vi "Merge Two Images.vi"(2 "Set Background Color (T)":bool=TRUE, 4 "Image 2 Bounds":T1={"Left"=0, "Top"=0, "Right"=64, "Bottom"=64}, 5 "Image 2 Data":T2, 6 "Image 1 Bounds":T1={"Left"=0, "Top"=0, "Right"=64, "Bottom"=64}, 7 "Image 1 Data":T2, 8 "error in (no error)":errorcluster, 9 "Background Color":u32(colorbox)=16777215, 10 "Image 2 Path":path, 11 "Image 1 Path":path) -> (0 "error out":errorcluster, 3 "Merged Image Data":T2)   [LabVIEW 2015]
doc: "This VI will merge two images into one. This merge supports PNGs and GIFs with alpha layers. Provide the path to <B>Image 1 Path</B> and <B>Image 2 Path</B> or provide the <B>Image 1 Data</B> and <B>Image 2 Data</B> or a combination of the two. Then provide the scaled <B>Image Bounds</B> and <B>Image 2 Bounds</B>. The output image will be large enough to contain both images. If both images have an alpha layer, then the <B>Background Color</B> should be provided.\n\n-------------\nDeveloped by Brian Hoover (hooovahh)"
uses:
  <vilib>/picture/picture.llb/imagedata.ctl
  <vilib>/Utility/miscctls.llb/LVRectTypeDef.ctl
  System.Drawing
  <vilib>/wsapi/NI_WebServices.lvlib
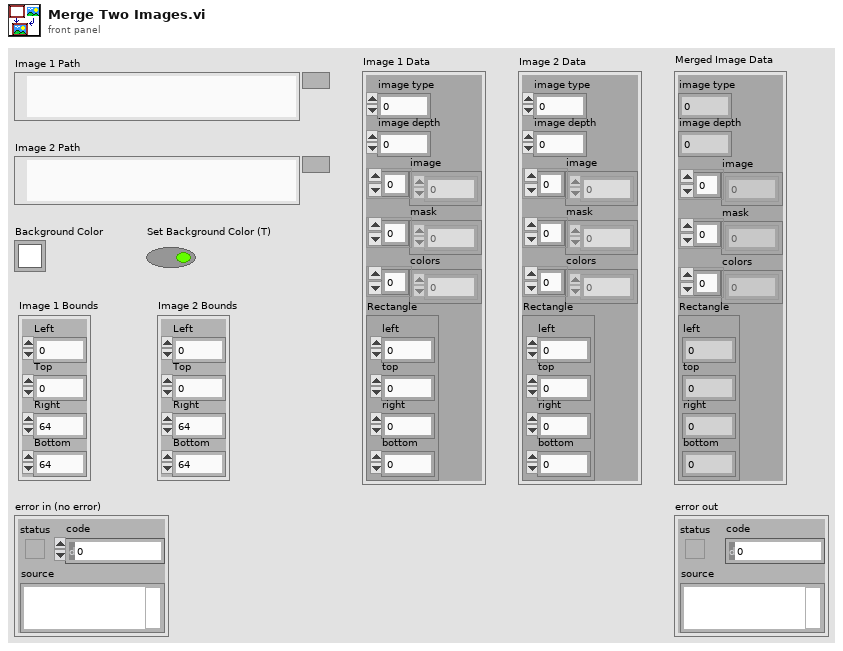
[diagram p1: front panel]
types:
  T1 = typedef "LVRectTypeDef.ctl" = cluster{"Left":i16, "Top":i16, "Right":i16, "Bottom":i16}
  T2 = typedef "imagedata.ctl" = cluster{"image type":i32, "image depth":i32, "image":u8[], "mask":u8[], "colors":u32[], "Rectangle":cluster{"left":i16, "top":i16, "right":i16, "bottom":i16}}
  T3 = typedef "LVBoundsTypeDef.ctl" = cluster{"Width":u32, "Height":u32}
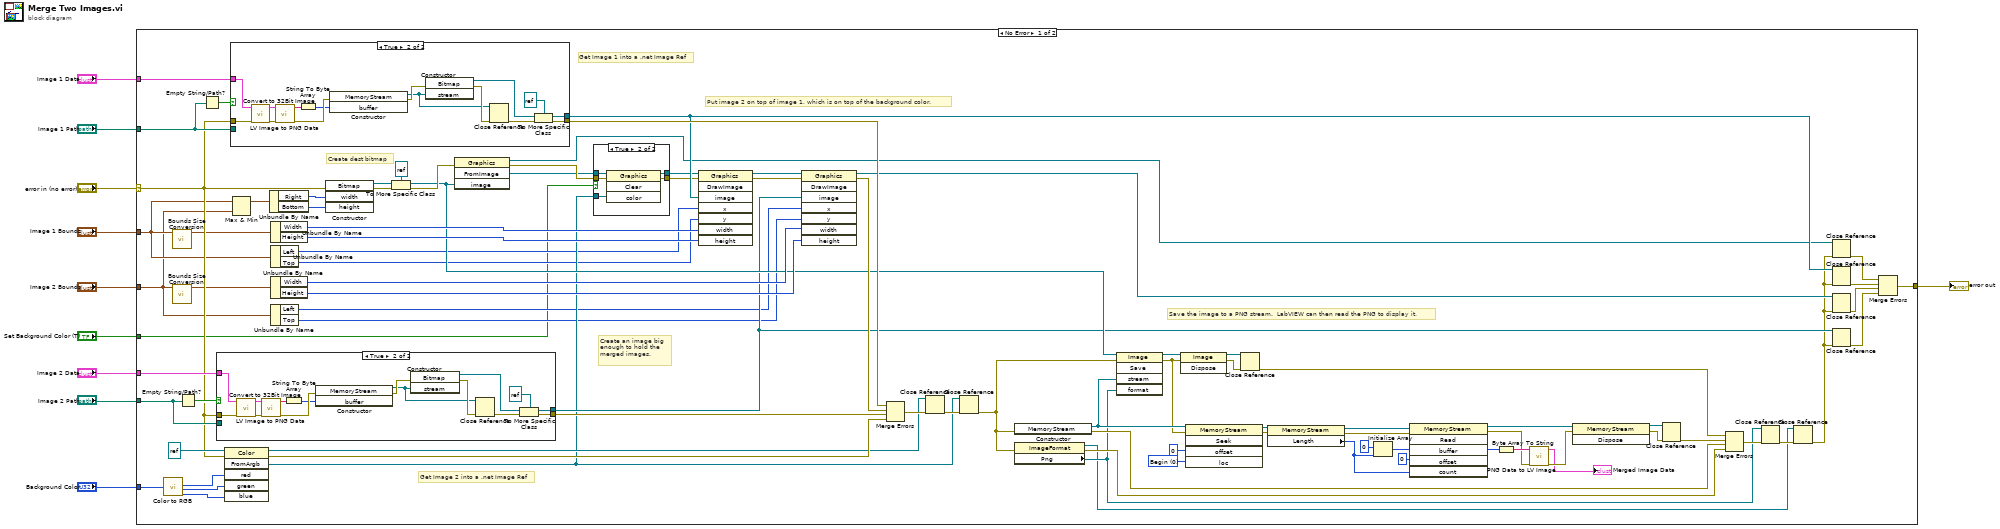
[diagram p0: block diagram]
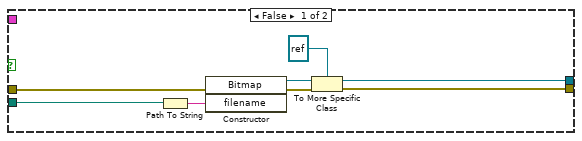
[diagram p3: hidden frame]
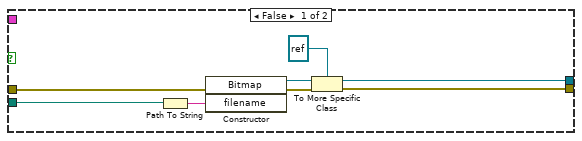
[diagram p4: hidden frame]
diagram:
  n1 = case shown="No Error" "error in (no error)" {
    selector: "error in (no error)" -> [w21 w153]
    tunnel: [w77 w153] -> w10
    tunnel: "Background Color" -> [w46 _]
    tunnel: "Image 1 Path" -> [w42 _]
    tunnel: "Image 1 Data" -> [w40 _]
    tunnel: "Image 2 Path" -> [w37 _]
    tunnel: "Image 2 Data" -> [w36 _]
    tunnel: "Image 1 Bounds" -> [w14 _]
    tunnel: "Image 2 Bounds" -> [w13 _]
    tunnel: "Set Background Color (T)" -> [w11 _]
    frame No Error {
      w69 = 0 items=["Begin", "Current", "End"] ("loc")
      # "Save the image to a PNG stream.  LabVIEW can then read the PNG to display it."
      # "Put image 2 on top of image 1, which is on top of the background color."
      # "Create an image big enough to hold the merged images."
      # "Get Image 1 into a .net Image Ref"
      # "Get Image 2 into a .net Image Ref"
      # "Create dest bitmap"
      n2 = call <vilib>:"Color to RGB.vi"("Color"=w46) -> ("R"=w45:u8, "G"=w44:u8, "B"=w43:u8)  [unwired: 1 out]
      n3 = call "Bounds Size Conversion.vi"("Bounds"=w14) -> ("Size Out"=w19:T3)  [unwired: 9 in, 1 out]
      n4 = call "Bounds Size Conversion.vi"("Bounds"=w13) -> ("Size Out"=w20:T3)  [unwired: 9 in, 1 out]
      n5 = Empty String/Path?(string/path=w37) -> (empty?=w38:bool)
      n6 = Empty String/Path?(string/path=w42) -> (empty?=w41:bool)
      n7 = case shown="True" w38 {
        tunnel: w21 -> [w110 w124]
        tunnel: w37 -> [w109 _]
        tunnel: [w108 w118] -> w35
        tunnel: [w107 w116] -> w39
        tunnel: w36 -> [_ w123]
        frame False {
          n8 = Path To String(path=w109) -> (string=w114:string)
          n9 = constructor class="Bitmap"(error in=w110, "filename"=w114) -> (reference out=w112:refnum<k24>, error out=w111:errorcluster)  [unwired: 2 in, 2 out]
          n10 = To More Specific Class(target class=refnum<k24> refnum, reference=w112, error in=w111) -> (specific class reference=w107:refnum<k24>, error out=w108:errorcluster)
        }
        frame True {
          n11 = call "Convert to 32Bit Image.vi"("error in (no error)"=w124, "Image Data"=w123) -> ("error out"=w125:errorcluster, "32Bit Image Data Out"=w126:T2)  [unwired: 8 in]
          n12 = call <vilib>:"LV Image to PNG Data.vi"("error in (no error)"=w125, "image data"=w126) -> ("error out"=w129:errorcluster, "png data"=w127:string)  [unwired: 8 in]
          n13 = String To Byte Array(string=w127) -> (unsigned byte array=w128:u8[])
          n14 = constructor class="MemoryStream"(error in=w129, "buffer"=w128) -> (reference out=w119:refnum<k24>, error out=w121:errorcluster)  [unwired: 2 in, 2 out]
          n15 = constructor class="Bitmap"(error in=w121, "stream"=w119) -> (reference out=w117:refnum<k24>, error out=w122:errorcluster)  [unwired: 2 in, 2 out]
          n16 = Close Reference(reference=w119, error in (no error)=w122) -> (error out=w120:errorcluster)
          n17 = To More Specific Class(target class=refnum<k24> refnum, reference=w117, error in=w120) -> (specific class reference=w116:refnum<k24>, error out=w118:errorcluster)
        }
      }
      n18 = invoke class="Color" method="FromArgb"(reference=refnum<k24> refnum ("color"), error in=w21, "red"=w45, "green"=w44, "blue"=w43) -> (reference out=w31:refnum<k24>, error out=w34:errorcluster, "FromArgb"=w29:refnum<k24>)  [unwired: 1 in, 3 out]
      n19 = case shown="True" w41 {
        tunnel: w21 -> [w133 w147]
        tunnel: w42 -> [w132 _]
        tunnel: [w131 w141] -> w94
        tunnel: [w130 w139] -> w93
        tunnel: w40 -> [_ w146]
        frame False {
          n20 = Path To String(path=w132) -> (string=w137:string)
          n21 = constructor class="Bitmap"(error in=w133, "filename"=w137) -> (reference out=w135:refnum<k24>, error out=w134:errorcluster)  [unwired: 2 in, 2 out]
          n22 = To More Specific Class(target class=refnum<k24> refnum, reference=w135, error in=w134) -> (specific class reference=w130:refnum<k24>, error out=w131:errorcluster)
        }
        frame True {
          n23 = call "Convert to 32Bit Image.vi"("error in (no error)"=w147, "Image Data"=w146) -> ("error out"=w148:errorcluster, "32Bit Image Data Out"=w149:T2)  [unwired: 8 in]
          n24 = call <vilib>:"LV Image to PNG Data.vi"("error in (no error)"=w148, "image data"=w149) -> ("error out"=w152:errorcluster, "png data"=w150:string)  [unwired: 8 in]
          n25 = String To Byte Array(string=w150) -> (unsigned byte array=w151:u8[])
          n26 = constructor class="MemoryStream"(error in=w152, "buffer"=w151) -> (reference out=w142:refnum<k24>, error out=w144:errorcluster)  [unwired: 2 in, 2 out]
          n27 = constructor class="Bitmap"(error in=w144, "stream"=w142) -> (reference out=w140:refnum<k24>, error out=w145:errorcluster)  [unwired: 2 in, 2 out]
          n28 = Close Reference(reference=w142, error in (no error)=w145) -> (error out=w143:errorcluster)
          n29 = To More Specific Class(target class=refnum<k24> refnum, reference=w140, error in=w143) -> (specific class reference=w139:refnum<k24>, error out=w141:errorcluster)
        }
      }
      n30 = Max & Min(x=w14, y=w13) -> (max(x,y)=w82:T1)  [unwired: 1 out]
      n31 = Unbundle By Name(w82) -> ("Right"=w84:i16, "Bottom"=w83:i16)
      n32 = Unbundle By Name(w19) -> ("Width"=w81:u32, "Height"=w79:u32)
      n33 = Unbundle By Name(w14) -> ("Left"=w18:i16, "Top"=w17:i16)
      n34 = Unbundle By Name(w20) -> ("Width"=w80:u32, "Height"=w78:u32)
      n35 = Unbundle By Name(w13) -> ("Left"=w16:i16, "Top"=w15:i16)
      n36 = constructor class="Bitmap"(error in=w21, "width"=w84, "height"=w83) -> (reference out=w98:refnum<k24>, error out=w97:errorcluster)  [unwired: 2 in, 3 out]
      n37 = To More Specific Class(target class=refnum<k24> refnum, reference=w98, error in=w97) -> (specific class reference=w76:refnum<k24>, error out=w96:errorcluster)
      n38 = invoke class="Graphics" method="FromImage"(error in=w96, "image"=w76) -> (reference out=w12:refnum<k24>, error out=w95:errorcluster, "FromImage"=w49:refnum<k24>)  [unwired: 2 in, 1 out]
      n39 = case shown="True" w11 {
        tunnel: w95 -> [w100 w106]
        tunnel: [w100 w105] -> w50
        tunnel: w49 -> [w101 w104]
        tunnel: [w101 w103] -> w48
        tunnel: w29 -> [_ w102]
        frame False {
        }
        frame True {
          n40 = invoke class="Graphics" method="Clear"(reference=w104, error in=w106, "color"=w102) -> (reference out=w103:refnum<k24>, error out=w105:errorcluster)  [unwired: 1 in, 2 out]
        }
      }
      n41 = invoke class="Graphics" method="DrawImage"(reference=w48, error in=w50, "image"=w93, "x"=w18, "y"=w17, "width"=w81, "height"=w79) -> (reference out=w89:refnum<k24>, error out=w90:errorcluster)  [unwired: 1 in, 6 out]
      n42 = invoke class="Graphics" method="DrawImage"(reference=w89, error in=w90, "image"=w39, "x"=w16, "y"=w15, "width"=w80, "height"=w78) -> (reference out=w88:refnum<k24>, error out=w87:errorcluster)  [unwired: 1 in, 6 out]
      n43 = Merge Errors(w94, w87, w35, w34) -> (w33:errorcluster)
      n44 = Close Reference(reference=w31, error in (no error)=w33) -> (error out=w32:errorcluster)
      n45 = Close Reference(reference=w29, error in (no error)=w32) -> (error out=w30:errorcluster)
      n46 = constructor class="MemoryStream"(error in=w30) -> (reference out=w55:refnum<k24>, error out=w27:errorcluster)  [unwired: 2 in, 1 out]
      n47 = property class="ImageFormat"(error in=w30) -> (reference out=w22:refnum<k24>, error out=w26:errorcluster, "Png"=w23:refnum<k24>)  [unwired: 1 in]
      n48 = invoke class="Image" method="Save"(reference=w76, error in=w30, "stream"=w55, "format"=w23) -> (reference out=w73:refnum<k24>, error out=w54:errorcluster)  [unwired: 1 in, 3 out]
      n49 = invoke class="Image" method="Dispose"(reference=w73, error in=w54) -> (reference out=w75:refnum<k24>, error out=w74:errorcluster)  [unwired: 1 in, 1 out]
      n50 = invoke class="MemoryStream" method="Seek"(reference=w55, error in=w54, "offset"=i64 0, "loc"=w69) -> (reference out=w72:refnum<k24>, error out=w71:errorcluster)  [unwired: 1 in, 3 out]
      n51 = Close Reference(reference=w75, error in (no error)=w74) -> (error out=w28:errorcluster)
      n52 = property class="MemoryStream"(reference=w72, error in=w71) -> (reference out=w67:refnum<k24>, error out=w66:errorcluster, "Length"=w64:i64)
      n53 = Initialize Array(u8 0 ("element"), w64) -> (w65:u8[])
      n54 = invoke class="MemoryStream" method="Read"(reference=w67, error in=w66, "buffer"=w65, "offset"=0, "count"=w64) -> (reference out=w62:refnum<k24>, error out=w58:errorcluster, "buffer"=w61:u8[])  [unwired: 1 in, 3 out]
      n55 = Byte Array To String(unsigned byte array=w61) -> (string=w60:string)
      n56 = call <vilib>:"PNG Data to LV Image.vi"("error in (no error)"=w58, "png data"=w60) -> ("error out"=w57:errorcluster, "image data"=→"Merged Image Data":T2)  [unwired: 8 in]
      n57 = invoke class="MemoryStream" method="Dispose"(reference=w62, error in=w57) -> (reference out=w59:refnum<k24>, error out=w56:errorcluster)  [unwired: 1 in, 1 out]
      n58 = Close Reference(reference=w59, error in (no error)=w56) -> (error out=w51:errorcluster)
      n59 = Merge Errors(w28, w51, w27, w26) -> (w52:errorcluster)
      n60 = Close Reference(reference=w23, error in (no error)=w52) -> (error out=w25:errorcluster)
      n61 = Close Reference(reference=w22, error in (no error)=w25) -> (error out=w24:errorcluster)
      n62 = Close Reference(reference=w12, error in (no error)=w24) -> (error out=w85:errorcluster)
      n63 = Close Reference(reference=w93, error in (no error)=w24) -> (error out=w92:errorcluster)
      n64 = Close Reference(reference=w88, error in (no error)=w24) -> (error out=w91:errorcluster)
      n65 = Close Reference(reference=w39, error in (no error)=w24) -> (error out=w86:errorcluster)
      n66 = Merge Errors(w85, w92, w91, w86) -> (w77:errorcluster)
    }
    frame Error {
    }
  }
  "error out" <- w10
